vi "calirbateList.vi"(8 "error in (no error)":errorcluster, 11 "ScriptEventList in":refnum<class "ScriptEventList.lvclass">) -> (0 "error out":errorcluster, 3 "ScriptEventList out":refnum<class "ScriptEventList.lvclass">)   [LabVIEW 2009, in "Tools.lvlib" / "Scripting.lvlib" / "ScriptEventList.lvclass"]
uses:
  ScriptEventList.lvclass
  ScriptEventList.lvclass/ScriptEventList.ctl
  ScriptEvent.lvclass
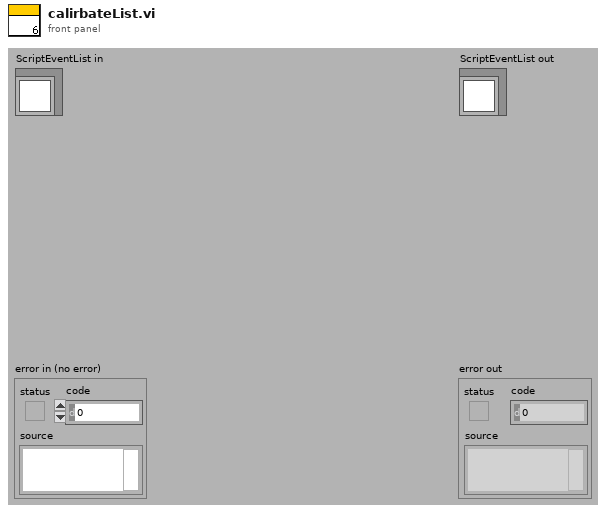
[diagram p1: front panel]
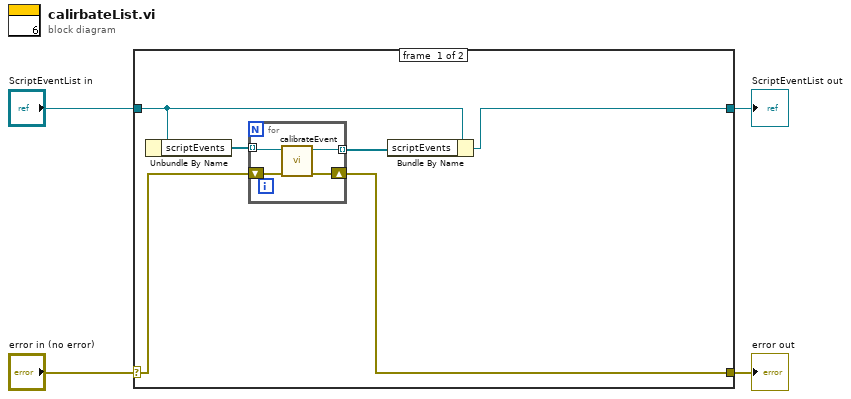
[diagram p0: block diagram]
diagram:
  n1 = case shown="No Error" "error in (no error)" {
    selector: "error in (no error)" -> [w9 w16]
    tunnel: [w8 w16] -> w3
    tunnel: [w5 w15] -> w1
    tunnel: "ScriptEventList in" -> [w6 w15]
    frame #0 {
      n2 = Unbundle By Name(w6) -> ("scriptEvents"=w10:refnum<class "ScriptEvent.lvclass">[])
      n3 = for {
        tunnel: w10 -> [w14] mode=indexing
        tunnel: [w13] -> w7 mode=indexing
        shift-right: [w11] -> w8
        shift-left: w9 -> [w12]
        n4 = call-dynamic "calibrateEvent.vi"("error in (no error)"=w12, "ScriptEvent in"=w14) -> ("error out"=w11:errorcluster, "ScriptEvent out"=w13:refnum<class "ScriptEvent.lvclass">)  [unwired: 8 in]
      }
      n5 = Bundle By Name(cluster=w6, "scriptEvents"=w7) -> (w5:refnum<class "ScriptEventList.lvclass">)
    }
    frame #1 {
    }
  }
  "error out" <- w3
  "ScriptEventList out" <- w1
